vi "Active_Target.vi"(9 "Session":u32, 10 "XYGraph Refnum":refnum<vi>) -> (0 "y0":dbl, 1 "x0":dbl, 2 "Active Plot":u32, 3 "Radius":dbl)   [LabVIEW 2010]
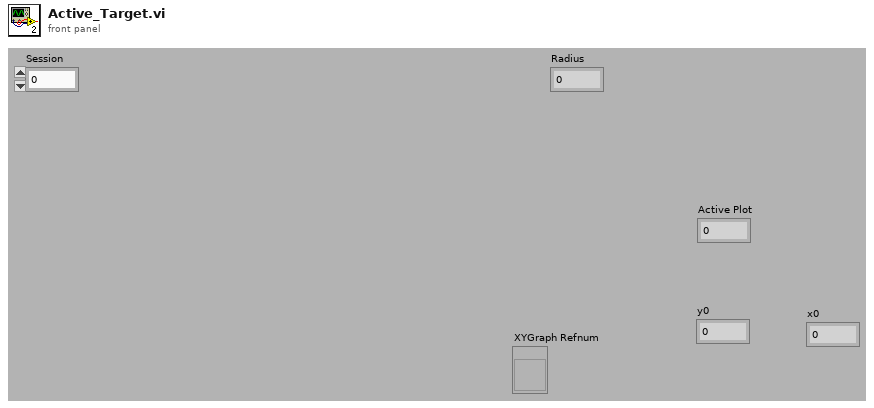
[diagram p1: front panel]
types:
  T1 = cluster{"Radius":dbl, "Center":dbl, "D":dbl, "Valid":bool}
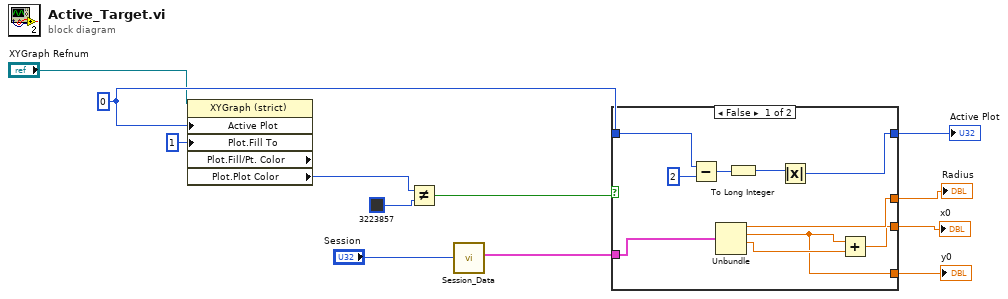
[diagram p0: block diagram]
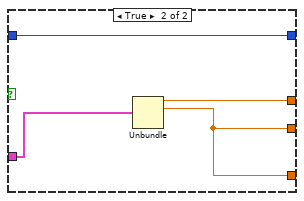
[diagram p2: hidden frame]
diagram:
  w10 = u32 0 ("Active Plot")
  n1 = property on="Property Node" class="XYGraph (strict)" props=["Active Plot", "Plot", "Fill To", "Plot", "Fill/Pt. Color", "Plot", "Plot Color"](reference="XYGraph Refnum", "Active Plot"=w10, "Plot.Fill To"=i16 1) -> ("Plot.Plot Color"=w7:u32)  [unwired: 1 in, 3 out]
  n2 = Not Equal?(x=w7, y=u32 3223857) -> (x != y?=w9:bool)
  n3 = call "Session_Data.vi"("Session"="Session") -> ("output cluster"=w4:T1)  [unwired: 10 in]
  n4 = case shown="False" w9 {
    tunnel: w10 -> [w22 w26]
    tunnel: [w18 w26] -> w11
    tunnel: w4 -> [w17 w25]
    tunnel: [w16 w24] -> w3
    tunnel: [w14 w23] -> w2
    tunnel: [w13 w23] -> w1
    frame False {
      n5 = Subtract(x=w22, y=u32 2) -> (x-y=w20:u32)
      n6 = Unbundle(w17) -> ("Radius"=w16:dbl, "Center"=w13:dbl, "D"=w15:dbl)  [unwired: 1 out]
      n7 = To Long Integer(number=w20) -> (32bit integer=w19:i32)
      n8 = Absolute Value(x=w19) -> (abs(x)=w18:i32)
      n9 = Add(x=w13, y=w15) -> (x+y=w14:dbl)
    }
    frame True {
      n10 = Unbundle(w25) -> ("Radius"=w24:dbl, "Center"=w23:dbl)  [unwired: 2 out]
    }
  }
  "Active Plot" <- w11
  "x0" <- w2
  "y0" <- w1
  "Radius" <- w3
